vi "Path as Encoded Path (LabVIEW Path).vi"(6 "error in":errorcluster, 9 "Path":path) -> (1 "Encoded Path":T1, 4 "error out":errorcluster)   [LabVIEW 2020, in "G-Unicode.lvlib"]
doc: "Converts the input path to a raw UTF-8 encoded LabVIEW path. Valid inputs are a UTF-8 Path class or LabVIEW path."
uses:
  G-Unicode.lvlib
  Types/Encoded UTF-8 Path.ctl
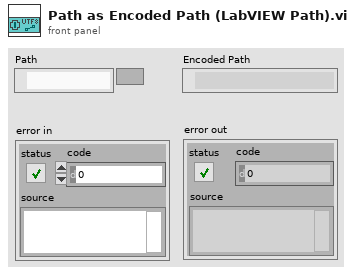
[diagram p1: front panel]
types:
  T1 = typedef "G-Unicode.lvlib/Encoded UTF-8 Path.ctl" = path
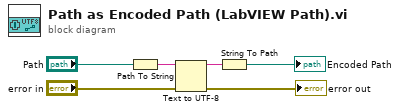
[diagram p0: block diagram]
diagram:
  n1 = Path To String(path="Path") -> (string=w1:string)
  n2 = Text to UTF-8(8:"error in", 11:w1) -> (0:→"error out":errorcluster, 3:w2:string)  [unwired: 1 in]
  n3 = String To Path(string=w2) -> (path=→"Encoded Path":path)
